vi "J1939 Data Lookup Table Set Signals (Range).vi"(8 "error in (no error)":errorcluster, 9 "Signals":dbl[](array[numeric]), 10 "Direct Access":cluster{"Offset":u32, "Length":u32}, 11 "Ref in":T1) -> (0 "error out":errorcluster {"code" min=0 max=0}, 3 "vi reference":T1)   [LabVIEW 2013, in "J1939.lvlib"]
uses:
  J1939.lvlib
  J1939 Data Lookup Table Reference.ctl
  J1939 Data Lookup Table Action.ctl
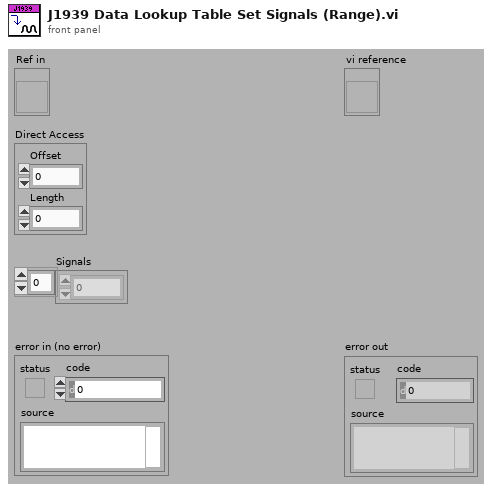
[diagram p1: front panel]
types:
  T1 = typedef "J1939.lvlib/J1939 Data Lookup Table Reference.ctl" = refnum<vi>
  T2 = typedef "J1939.lvlib/J1939 Data Lookup Table Action.ctl" = enum16{"Get All", "Set All", "Set Frame", "Get Frame", "Set Range", "Get Range"}
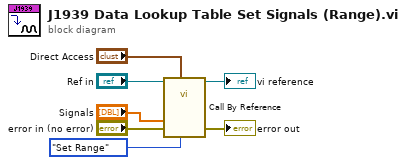
[diagram p0: block diagram]
diagram:
  n1 = call-by-ref "?"(reference="Ref in", "command"=J1939_Data_Lookup_Table_Action."Set Range", "Direct Access"="Direct Access", "error in (no error)"="error in (no error)", "Signals"="Signals") -> (reference out=→"vi reference":T1, "error out"=→"error out":errorcluster)  [unwired: 7 in, 2 out]
